vi "Test INI file.vi"() -> ()   [LabVIEW 2018]
uses:
  <vilib>/Utility/config.llb/Read Key (String).vi
  <vilib>/Utility/config.llb/NI_LVConfig.lvlib
  <vilib>/Utility/config.llb/Write Key (Double).vi
panel:
  out "section":string[](array[string])
  out "Key Value":string[][](array[string])
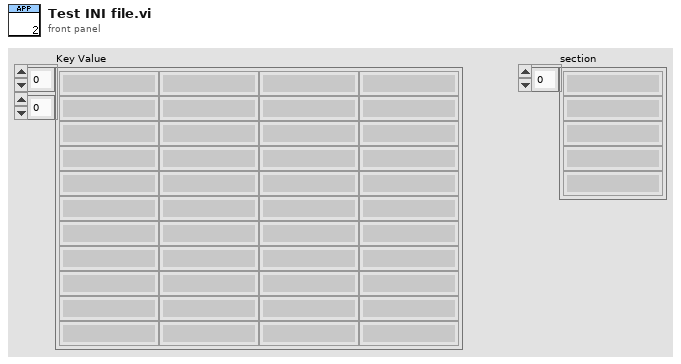
[diagram p1: front panel]
types:
  T1 = typedef "NI_LVConfig.lvlib/Config Data RefNum.ctl" = refnum<k1>
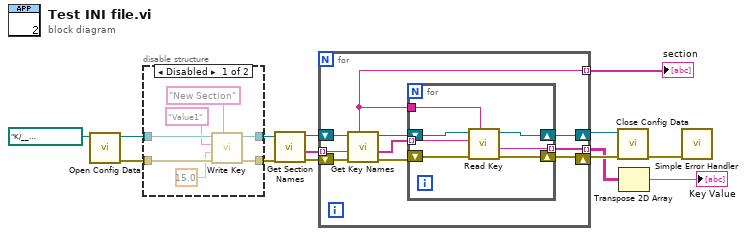
[diagram p0: block diagram]
diagram:
  n1 = call <vilib>:"Open Config Data.vi"("configuration file path"=path "K:/__RangDongCorp(thay tcuong,cHanh)/Technical Solution/software/lv_apps_v3/HV-60D_LVapps/HV-60D.INI") -> ("error out"=w3:errorcluster, "refnum"=w4:T1)  [unwired: 8 in, 1 out]
  n2 = disable-structure shown="Disabled" {
    disable-tunnel: w4 -> [w21 w23]
    disable-tunnel: w3 -> [w20 w22]
    disable-tunnel: [w16 w22] -> w2
    disable-tunnel: [w15 w23] -> w1
    frame Disabled {
      n3 = call-poly <vilib>:"Write Key.vi"("section"="New Section", "error in (no error)"=w20, "value"=15.0, "key"="Value1", "refnum"=w21) -> ("error out"=w16:errorcluster, "refnum out"=w15:T1)  [unwired: 4 in, 1 out]
    }
    frame Enabled {
    }
  }
  n4 = call <vilib>:"Get Section Names.vi"("error in (no error)"=w2, "refnum"=w1) -> ("error out"=w11:errorcluster, "section names"=w13:string[], "refnum out"=w12:T1)  [unwired: 7 in]
  n5 = for {
    tunnel: w13 -> [w24] mode=indexing
    shift-right: [w28] -> w10
    shift-left: w12 -> [w32]
    tunnel: [w29] -> w6 mode=indexing
    shift-right: [w25] -> w9
    shift-left: w11 -> [w26]
    tunnel: [w24] -> w7 mode=indexing
    n6 = call <vilib>:"Get Key Names.vi"("section"=w24, "error in (no error)"=w26, "refnum"=w32) -> ("error out"=w27:errorcluster, "key names"=w31:string[], "refnum out"=w30:T1)  [unwired: 5 in, 1 out]
    n7 = for {
      tunnel: w31 -> [w36] mode=indexing
      shift-right: [w38] -> w28
      shift-left: w30 -> [w39]
      tunnel: w24 -> [w37]
      tunnel: [w35] -> w29 mode=indexing
      shift-right: [w34] -> w25
      shift-left: w27 -> [w33]
      n8 = call-poly <vilib>:"Read Key.vi"("section"=w37, "error in (no error)"=w33, "key"=w36, "refnum"=w39) -> ("error out"=w34:errorcluster, "value"=w35:string, "refnum out"=w38:T1)  [unwired: 4 in, 1 out]
    }
  }
  "section" <- w7
  n9 = call <vilib>:"Close Config Data.vi"("error in (no error)"=w9, "refnum"=w10) -> ("error out"=w8:errorcluster)  [unwired: 8 in, 1 out]
  n10 = Transpose 2D Array(2D array=w6) -> (transposed array=→"Key Value":string[][])
  n11 = call <vilib>:"Simple Error Handler.vi"("error in (no error)"=w8) -> ()  [unwired: 4 in, 5 out]
